vi "SEPXP [Event Registration Refnum] to Cluster.vi"(11 "Tipstrips Event Registrations":refnum<event-registration>[](array[refnum])) -> (3 "Tipstrip RE refnums":T1)   [LabVIEW 2019]
uses:
  SEPXP Tipstrip Event Registration Refnums.ctl
  XY Graph Refnum.ctl
  XY Graph Add-Ons.lvlib
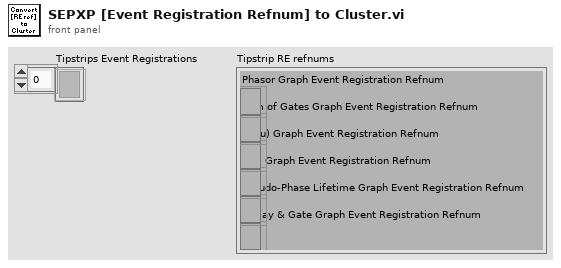
[diagram p1: front panel]
types:
  T1 = typedef "SEPXP Tipstrip Event Registration Refnums.ctl" = cluster{"Phasor Graph Event Registration Refnum":refnum<event-registration>, "Sum of Gates Graph Event Registration Refnum":refnum<event-registration>, "f(tau) Graph Event Registration Refnum":refnum<event-registration>, "a(b) Graph Event Registration Refnum":refnum<event-registration>, "Pseudo-Phase Lifetime Graph Event Registration Refnum":refnum<event-registration>, "Decay & Gate Graph Event Registration Refnum":refnum<event-registration>}
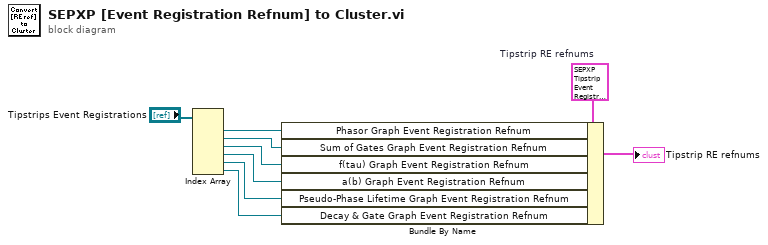
[diagram p0: block diagram]
diagram:
  w7 = T1 {"Phasor Graph Event Registration Refnum"=refnum, "Sum of Gates Graph Event Registration Refnum"=refnum, "f(tau) Graph Event Registration Refnum"=refnum, "a(b) Graph Event Registration Refnum"=refnum, "Pseudo-Phase Lifetime Graph Event Registration Refnum"=refnum, "Decay & Gate Graph Event Registration Refnum"=refnum}  # Tipstrip RE refnums
  n1 = Index Array(array="Tipstrips Event Registrations") -> (element #1=w8:refnum<event-registration>, element #2=w5:refnum<event-registration>, element #3=w4:refnum<event-registration>, element #4=w3:refnum<event-registration>, element #5=w2:refnum<event-registration>, element #6=w1:refnum<event-registration>)  [unwired: 6 in]
  n2 = Bundle By Name(cluster=w7, "Phasor Graph Event Registration Refnum"=w8, "Sum of Gates Graph Event Registration Refnum"=w5, "f(tau) Graph Event Registration Refnum"=w4, "a(b) Graph Event Registration Refnum"=w3, "Pseudo-Phase Lifetime Graph Event Registration Refnum"=w2, "Decay & Gate Graph Event Registration Refnum"=w1) -> (→"Tipstrip RE refnums":T1)
